vi "#152_MAV_MSG_MEMINFO_DECODE.vi"(11 "mavlink_payload":u8[](array[numeric])) -> (3 "MEMINFO":T1)   [LabVIEW 2023]
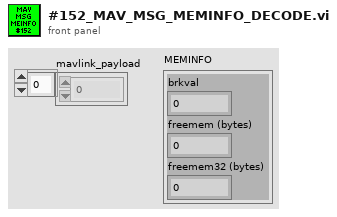
[diagram p1: front panel]
types:
  T1 = cluster{"brkval":u16, "freemem (bytes)":u16, "freemem32 (bytes)":u32}
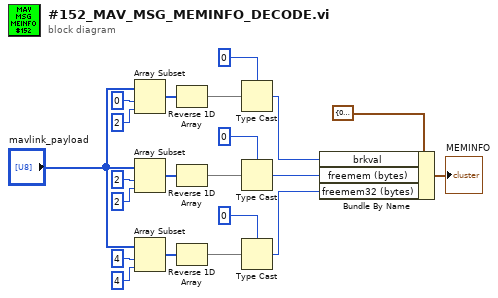
[diagram p0: block diagram]
diagram:
  n1 = Array Subset(array="mavlink_payload", index=0, length=2) -> (w21:u8[])
  n2 = Array Subset(array="mavlink_payload", index=2, length=2) -> (w13:u8[])
  n3 = Array Subset(array="mavlink_payload", index=4, length=4) -> (w7:u8[])
  n4 = Reverse 1D Array(array=w21) -> (reversed array=w20:u8[])
  n5 = Reverse 1D Array(array=w13) -> (reversed array=w12:u8[])
  n6 = Reverse 1D Array(array=w7) -> (reversed array=w6:u8[])
  n7 = Type Cast(type=u16 0 ("index"), x=w20) -> (*(type *) &x=w14:u16)
  n8 = Type Cast(type=u16 0 ("index"), x=w12) -> (*(type *) &x=w8:u16)
  n9 = Type Cast(type=u32 0 ("index"), x=w6) -> (*(type *) &x=w1:u32)
  n10 = Bundle By Name(cluster=T1 {"brkval"=0, "freemem (bytes)"=0, "freemem32 (bytes)"=0} ("MEMINFO"), "brkval"=w14, "freemem (bytes)"=w8, "freemem32 (bytes)"=w1) -> (→"MEMINFO":T1)
